vi "Read Configuration Data.vi"(8 "error in (no error)":errorcluster) -> (0 "error out":errorcluster, 3 "Cluster":T1)   [LabVIEW 2017]
uses:
  Configuration Data.ctl
  Car Wash System Globals.vi
  <vilib>/Utility/config.llb/NI_LVConfig.lvlib
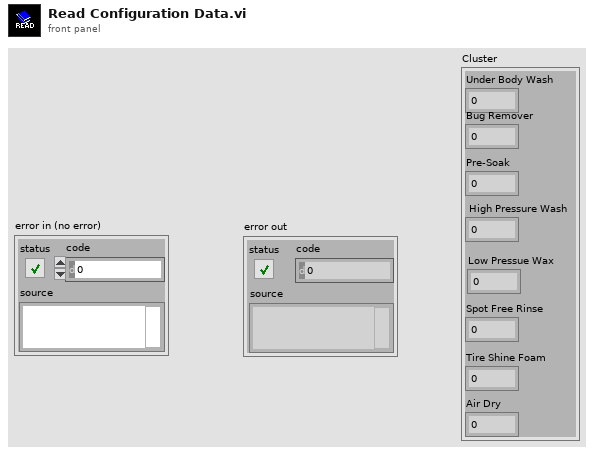
[diagram p1: front panel]
types:
  T1 = typedef "Configuration Data.ctl" = cluster{"Under Body Wash ":dbl, "Bug Remover":dbl, "Pre-Soak":dbl, " High Pressure Wash":dbl, "Low Pressue Wax ":dbl, "Spot Free Rinse ":dbl, "Tire Shine Foam":dbl, "Air Dry ":dbl}
  T2 = typedef "NI_LVConfig.lvlib/Config Data RefNum.ctl" = refnum<k1>
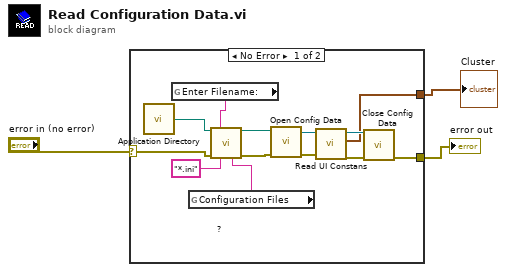
[diagram p0: block diagram]
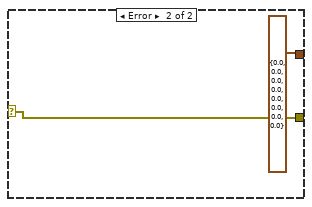
[diagram p2: hidden frame]
diagram:
  n1 = case shown="No Error" "error in (no error)" {
    selector: "error in (no error)" -> [w12 w18]
    tunnel: [w9 w18] -> w2
    tunnel: [w4 T1 {"Under Body Wash "=0.0, "Bug Remover"=0.0, "Pre-Soak"=0.0, " High Pressure Wash"=0.0, "Low Pressue Wax "=0.0, "Spot Free Rinse "=0.0, "Tire Shine Foam"=0.0, "Air Dry "=0.0} ("Condiguration Data")] -> w1
    frame No Error {
      n2 = call <vilib>:"Application Directory.vi"() -> ("Application Directory"=w14:path)
      n3 = global read "Car Wash System Globals.vi" "Enter Filename:"() -> (w15:string)
      n4 = global read "Car Wash System Globals.vi" "Configuration Files"() -> (w11:string)
      n5 = call "?"("start path"=w14, "prompt"=w15, "error in"=w12, "pattern (all files)"="*.ini", "pattern label"=w11) -> ("selected path"=w10:path, "error out"=w13:errorcluster)  [unwired: 7 in, 2 out]
      n6 = call <vilib>:"Open Config Data.vi"("error in (no error)"=w13, "configuration file path"=w10) -> ("error out"=w8:errorcluster, "refnum"=w7:T2)  [unwired: 7 in, 1 out]
      n7 = call "Read UI Constans.vi"("error in (no error)"=w8, "CFG File Refnum in"=w7) -> ("error out"=w5:errorcluster, "Cluster"=w4:T1, "CFG File Refnum out"=w6:T2)  [unwired: 7 in]
      n8 = call <vilib>:"Close Config Data.vi"("error in (no error)"=w5, "refnum"=w6) -> ("error out"=w9:errorcluster)  [unwired: 8 in, 1 out]
    }
    frame Error {
    }
  }
  "error out" <- w2
  "Cluster" <- w1
